vi "BRig_RT__Case_Exp__recordAnalogInput__PortA__fifo__1value__v2.vi"(2 "input_iOccurence":u16, 3 "resetOccurrence":bool, 4 "input_dataCurrent":u16[](array[numeric]), 5 "input_AnaIn_array":u16[][](array[numeric]), 6 "input_iState_start":T1, 7 "rt fifo":refnum<k33>, 8 "input_iState_end":T1, 9 "input_fifo_error":errorcluster) -> (11 "output_fifo_error":errorcluster, 13 "rt fifo out":refnum<k33>, 16 "output_iOccurrence":u16)   [LabVIEW 2014]
uses:
  myRIO_BRig_RT__Case_Exp_stateList.ctl
panel:
  out "anyTimeout":bool
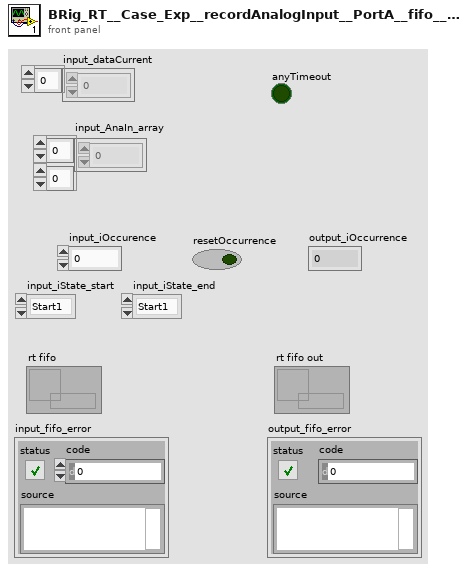
[diagram p1: front panel]
types:
  T1 = typedef "myRIO_BRig_RT__Case_Exp_stateList.ctl" = enum16{"Start1", "Start2", "Start3", "saveSettings1", "saveSettings2", "saveSettings3", "saveSettings4", "saveSettings_LC_ENL_l1", "saveSettings_LC_ENL_l2", "saveSettings_LC_Cue_l1", "saveSettings_LC_Cue_l2", "saveSettings6_LC_l1_Other", "SaveSettings6_LC_l2_Other", "setSettings_Audio", "setSettings_Laser", "initBlock_pre", "initBlock", "initBlock2", "initBlock_post", "initTrial_pre", "initTrial", "initTrial2", "initTrial3", "initTrial4", "initTrial_LC_ENL1", "initTrial_LC_Cue1", "initTrial_LC_Cue1_2", "initTrial_LC_Sel", "initTrial_post", "ENL1_pre", "ENL1", "ENL1_post", "ENL1Penalty_pre", "ENL1Penalty", "ENL2_pre", "ENL2", "ENL2Penalty_pre", "ENL2Penalty", "Cue1_pre", "Cue1", "Cue1_post", "Cue1Penalty_pre", "Cue1Penalty", "Cue2_pre", "Cue2", "Cue2Penalty_pre", "Cue2Penalty", "Selection_pre", "Selection", "Select_post", "SelectReward_pre", "SelectReward", "SelectRewardPost_pre", "SelectRewardPost", "SelectWrong_pre", "SelectWrong", "SelectWrong_post", "SelectTimeout_pre", "SelectTimeout", "SelectTimeout_post", "endTrial_pre", "endTrial1", "endTrial2", "endTrial3", "endTrial_post", "endBlock_pre", "endBlock", "endBlock_post", "endExp", "commConnect", "commUpload_pre", "commUpload_dataBlock", "commUpload_dataCurrent", "commUpload_dataExp", "commUpload_dataLC", "commUpload_dataTrial", "commUpload_post", "saveData_pre", "saveData_dataBlock", "saveData_dataCurrent", "saveData_dataExp", "saveData_dataLC", "saveData_dataTrial", "saveData_post", "empty_endBlock1", "empty_endBlock2", "empty_endTrial1", "empty_endTrial2", "empty_endTrial3", "empty_endTrial4", "empty_endTrial5", "dummyState", "dummyState_endBlock", "FreeReward_pre", "FreeReward", "FreeRewardPost_pre", "FreeRewardPost"}
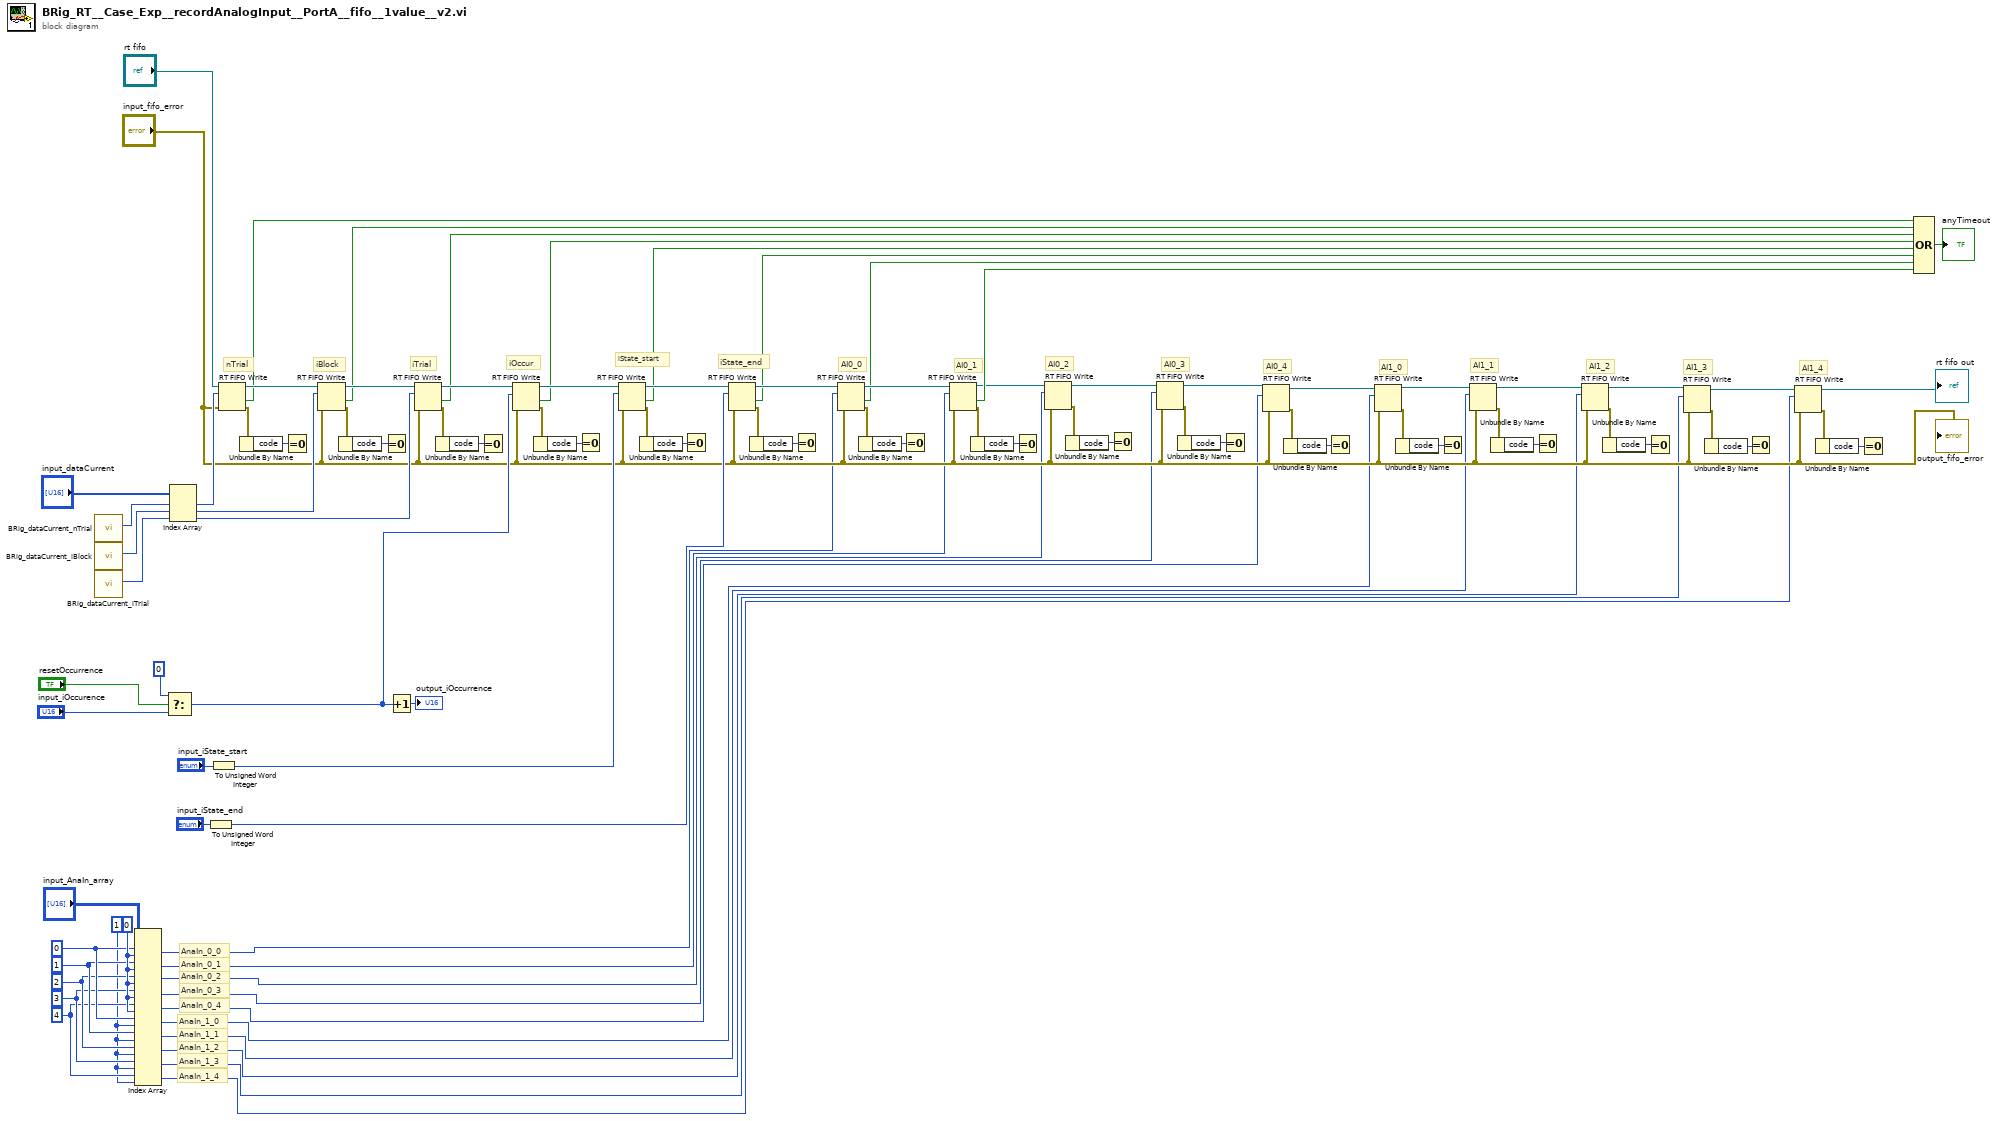
[diagram p0: block diagram]
diagram:
  w37 = 1 ("milliseconds to wait")
  w43 = 0 ("milliseconds to wait")
  w38 = 4 ("milliseconds to wait")
  w39 = 3 ("milliseconds to wait")
  w40 = 2 ("milliseconds to wait")
  w41 = 1 ("milliseconds to wait")
  w42 = 0 ("milliseconds to wait")
  # "AI1_4"
  # "AI1_3"
  # "AI1_2"
  # "AI1_1"
  # "AI1_0"
  # "AI0_4"
  # "AI0_3"
  # "AI0_2"
  # "AnaIn_1_4"
  # "AnaIn_1_3"
  # "AnaIn_1_2"
  # "AnaIn_1_1"
  # "AnaIn_1_0"
  # "AnaIn_0_4"
  # "AnaIn_0_3"
  # "AnaIn_0_2"
  # "AnaIn_0_1"
  # "AnaIn_0_0"
  # "AI0_1"
  # "AI0_0"
  # "iState_end"
  # "iState_start"
  # "iOccur"
  # "iTrial"
  # "iBlock"
  # "nTrial"
  n1 = call "BRig_dataCurrent_nTrial.vi"() -> ("output_nTrial"=w92:i32)  [unwired: 11 in]
  n2 = call "BRig_dataCurrent_iBlock.vi"() -> ("output_iBlock"=w91:i32)  [unwired: 11 in]
  n3 = call "BRig_dataCurrent_iTrial.vi"() -> ("output_iTrial"=w90:i32)  [unwired: 11 in]
  n4 = Index Array(array="input_AnaIn_array", index (row) #1=w42, index (col) #1=w43, index (row) #2=w41, index (col) #2=w43, index (row) #3=w40, index (col) #3=w43, index (row) #4=w39, index (col) #4=w43, index (row) #5=w38, index (col) #5=w43, index (row) #6=w42, index (col) #6=w37, index (row) #7=w41, index (col) #7=w37, index (row) #8=w40, index (col) #8=w37, index (row) #9=w39, index (col) #9=w37, index (row) #10=w38, index (col) #10=w37) -> (element #1=w10:u16, element #2=w9:u16, element #3=w8:u16, element #4=w7:u16, element #5=w6:u16, element #6=w5:u16, element #7=w4:u16, element #8=w3:u16, element #9=w2:u16, element #10=w1:u16)
  n5 = Select(t=u16 0, s="resetOccurrence", f="input_iOccurence") -> (s? t:f=w56:u16)
  n6 = Index Array(array="input_dataCurrent", index #1=w92, index #2=w91, index #3=w90) -> (element #1=w59:u16, element #2=w58:u16, element #3=w57:u16)
  n7 = To Unsigned Word Integer(number="input_iState_end") -> (unsigned 16bit integer=w54:u16)
  n8 = To Unsigned Word Integer(number="input_iState_start") -> (unsigned 16bit integer=w55:u16)
  n9 = RT FIFO Write(0:"rt fifo", 1:w59, 3:"input_fifo_error") -> (8:w77:refnum<k33>, 10:w46:bool, 11:w76:errorcluster)  [unwired: 2 in, 1 out]
  n10 = Unbundle By Name(w76) -> ("code"=w81:i32)
  n11 = Equal To 0?(x=w81) -> ()  [unwired: 1 out]
  n12 = RT FIFO Write(0:w77, 1:w58, 3:"input_fifo_error") -> (8:w73:refnum<k33>, 10:w47:bool, 11:w79:errorcluster)  [unwired: 2 in, 1 out]
  n13 = Unbundle By Name(w79) -> ("code"=w78:i32)
  n14 = Equal To 0?(x=w78) -> ()  [unwired: 1 out]
  n15 = Increment(x=w56) -> (x+1=→"output_iOccurrence":u16)
  n16 = RT FIFO Write(0:w73, 1:w57, 3:"input_fifo_error") -> (8:w70:refnum<k33>, 10:w48:bool, 11:w75:errorcluster)  [unwired: 2 in, 1 out]
  n17 = Unbundle By Name(w75) -> ("code"=w74:i32)
  n18 = Equal To 0?(x=w74) -> ()  [unwired: 1 out]
  n19 = RT FIFO Write(0:w70, 1:w56, 3:"input_fifo_error") -> (8:w67:refnum<k33>, 10:w49:bool, 11:w71:errorcluster)  [unwired: 2 in, 1 out]
  n20 = Unbundle By Name(w71) -> ("code"=w72:i32)
  n21 = Equal To 0?(x=w72) -> ()  [unwired: 1 out]
  n22 = RT FIFO Write(0:w67, 1:w55, 3:"input_fifo_error") -> (8:w64:refnum<k33>, 10:w50:bool, 11:w68:errorcluster)  [unwired: 2 in, 1 out]
  n23 = Unbundle By Name(w68) -> ("code"=w69:i32)
  n24 = Equal To 0?(x=w69) -> ()  [unwired: 1 out]
  n25 = RT FIFO Write(0:w64, 1:w54, 3:"input_fifo_error") -> (8:w61:refnum<k33>, 10:w51:bool, 11:w65:errorcluster)  [unwired: 2 in, 1 out]
  n26 = Unbundle By Name(w65) -> ("code"=w66:i32)
  n27 = Equal To 0?(x=w66) -> ()  [unwired: 1 out]
  n28 = RT FIFO Write(0:w61, 1:w10, 3:"input_fifo_error") -> (8:w60:refnum<k33>, 10:w52:bool, 11:w62:errorcluster)  [unwired: 2 in, 1 out]
  n29 = Unbundle By Name(w62) -> ("code"=w63:i32)
  n30 = Equal To 0?(x=w63) -> ()  [unwired: 1 out]
  n31 = RT FIFO Write(0:w60, 1:w9, 3:"input_fifo_error") -> (8:w31:refnum<k33>, 10:w53:bool, 11:w82:errorcluster)  [unwired: 2 in, 1 out]
  n32 = Unbundle By Name(w82) -> ("code"=w83:i32)
  n33 = Equal To 0?(x=w83) -> ()  [unwired: 1 out]
  n34 = RT FIFO Write(0:w31, 1:w8, 3:"input_fifo_error") -> (8:w32:refnum<k33>, 11:w33:errorcluster)  [unwired: 2 in, 2 out]
  n35 = Unbundle By Name(w33) -> ("code"=w34:i32)
  n36 = Equal To 0?(x=w34) -> ()  [unwired: 1 out]
  n37 = RT FIFO Write(0:w32, 1:w7, 3:"input_fifo_error") -> (8:w19:refnum<k33>, 11:w35:errorcluster)  [unwired: 2 in, 2 out]
  n38 = Unbundle By Name(w35) -> ("code"=w36:i32)
  n39 = Equal To 0?(x=w36) -> ()  [unwired: 1 out]
  n40 = RT FIFO Write(0:w19, 1:w6, 3:"input_fifo_error") -> (8:w26:refnum<k33>, 11:w27:errorcluster)  [unwired: 2 in, 2 out]
  n41 = Unbundle By Name(w27) -> ("code"=w28:i32)
  n42 = Equal To 0?(x=w28) -> ()  [unwired: 1 out]
  n43 = RT FIFO Write(0:w26, 1:w5, 3:"input_fifo_error") -> (8:w20:refnum<k33>, 11:w29:errorcluster)  [unwired: 2 in, 2 out]
  n44 = Unbundle By Name(w29) -> ("code"=w30:i32)
  n45 = Equal To 0?(x=w30) -> ()  [unwired: 1 out]
  n46 = RT FIFO Write(0:w20, 1:w4, 3:"input_fifo_error") -> (8:w21:refnum<k33>, 11:w22:errorcluster)  [unwired: 2 in, 2 out]
  n47 = Unbundle By Name(w22) -> ("code"=w23:i32)
  n48 = Equal To 0?(x=w23) -> ()  [unwired: 1 out]
  n49 = RT FIFO Write(0:w21, 1:w3, 3:"input_fifo_error") -> (8:w13:refnum<k33>, 11:w24:errorcluster)  [unwired: 2 in, 2 out]
  n50 = Unbundle By Name(w24) -> ("code"=w25:i32)
  n51 = Equal To 0?(x=w25) -> ()  [unwired: 1 out]
  n52 = RT FIFO Write(0:w13, 1:w2, 3:"input_fifo_error") -> (8:w14:refnum<k33>, 11:w15:errorcluster)  [unwired: 2 in, 2 out]
  n53 = Unbundle By Name(w15) -> ("code"=w16:i32)
  n54 = Equal To 0?(x=w16) -> ()  [unwired: 1 out]
  n55 = RT FIFO Write(0:w14, 1:w1, 3:"input_fifo_error") -> (8:→"rt fifo out":refnum<k33>, 11:w17:errorcluster)  [unwired: 2 in, 2 out]
  n56 = Unbundle By Name(w17) -> ("code"=w18:i32)
  n57 = Equal To 0?(x=w18) -> ()  [unwired: 1 out]
  n58 = Compound Arithmetic op=OR(w46, w47, w48, w49, w50, w51, w52, w53) -> (→"anyTimeout":bool)
  "output_fifo_error" <- "input_fifo_error"
